vi "MergeFilesManual.vi"(4 "Error In":errorcluster, 7 "MergeFileConfINPUT":T1) -> (0 "sortie d'erreur":errorcluster)   [LabVIEW 2017]
uses:
  DefDeType/MergeFileConfig.ctl
  DefDeType/WhichPath.ctl
panel:
  out "MergeFileConfig":T1
  in  "Cancel":bool
  in  "OK Merge":bool
  out "AllWaveForms":waveform(dbl)[](graph)
  out "QUALISYSWaveForms":waveform(dbl)[](graph)
  out "HBMWaveform":waveform(dbl)[](graph)
  out "PCIWaveforms":waveform(dbl)[](graph)
  out "Etat":string
  # "Merging files"
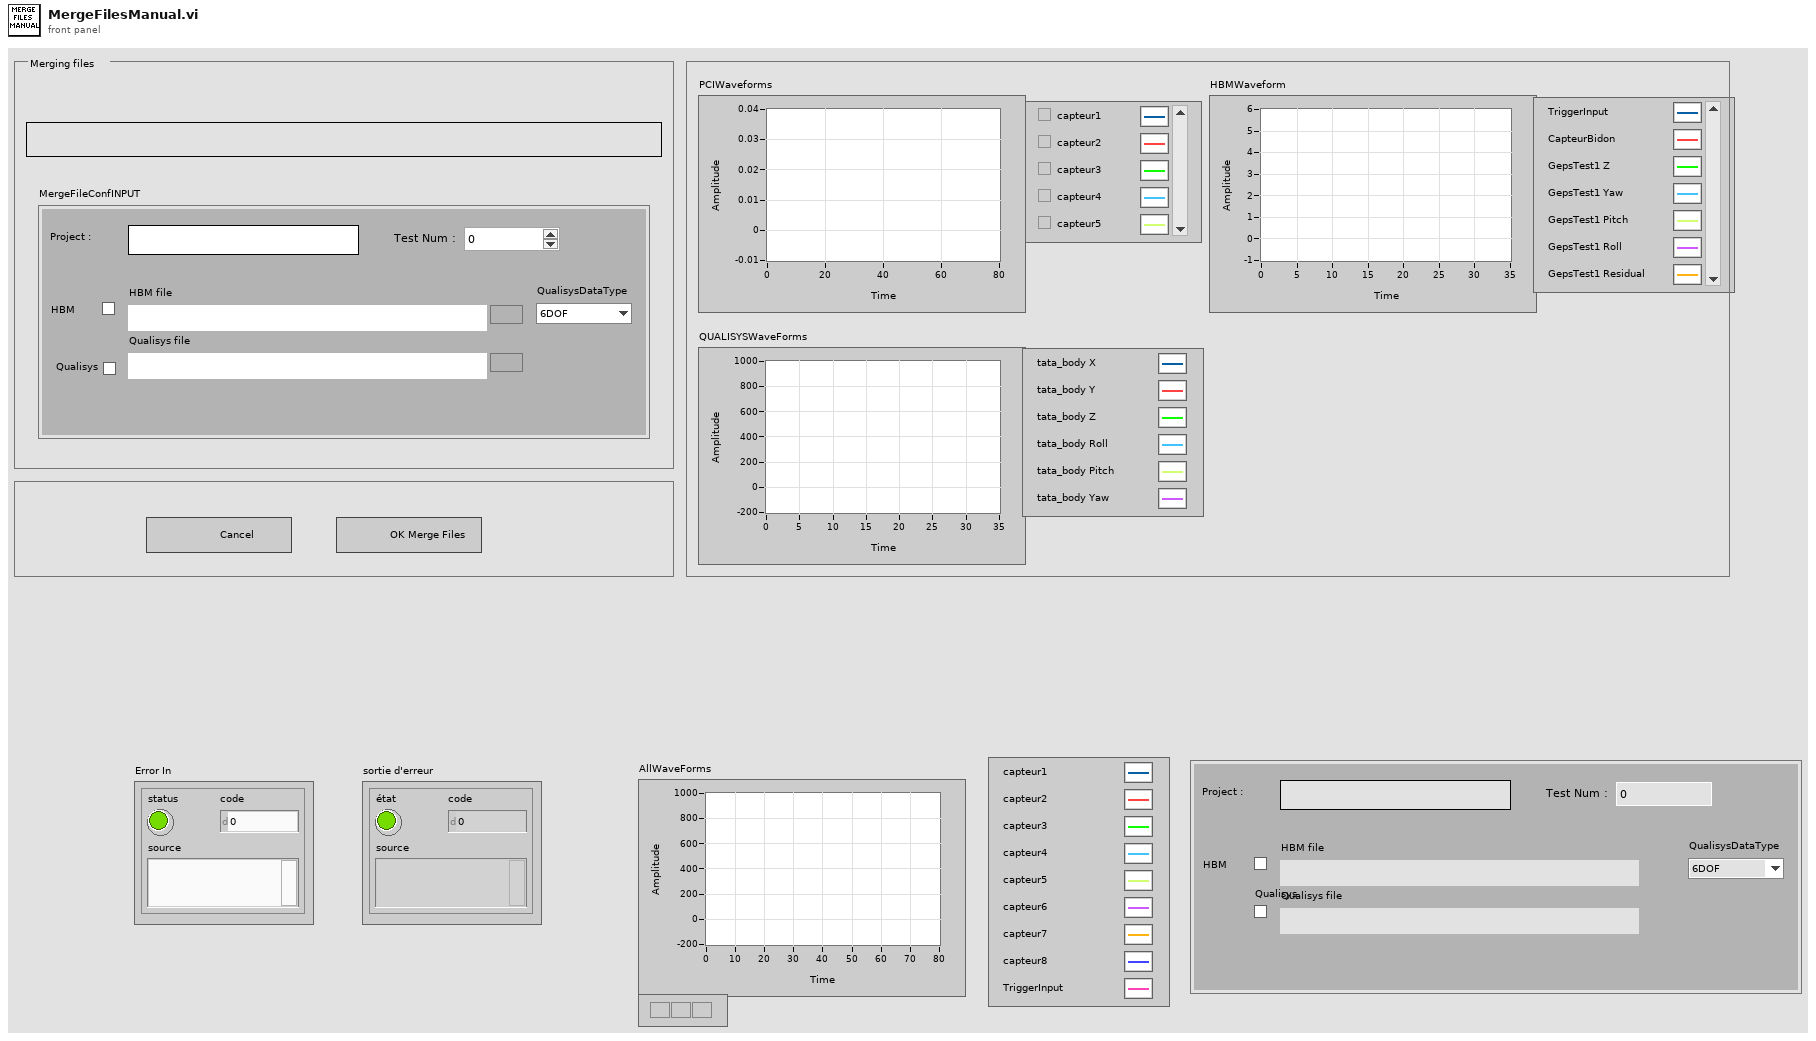
[diagram p1: front panel]
types:
  T1 = typedef "MergeFileConfig.ctl" = cluster{"Test Num : ":u32, "Project :":string, "Qualisys file":path, "HBM file":path, "QualisysDataType":enum16{"6DOF", "3DTracking", "6DOF + 3D"}, "Qualisys":bool, "HBM":bool}
  T2 = enum16{"open", "open or create", "create or replace", "create", "open (read-only)"}
  T3 = typedef "WhichPath.ctl" = enum16{"DossierProjet", "Config", "Meas", "MeasPCI", "MeasCRIO1", "MeasCRIO2", "MeasQualisys", "MeasHBM", "MeasTDMS", "Fig", "Res"}
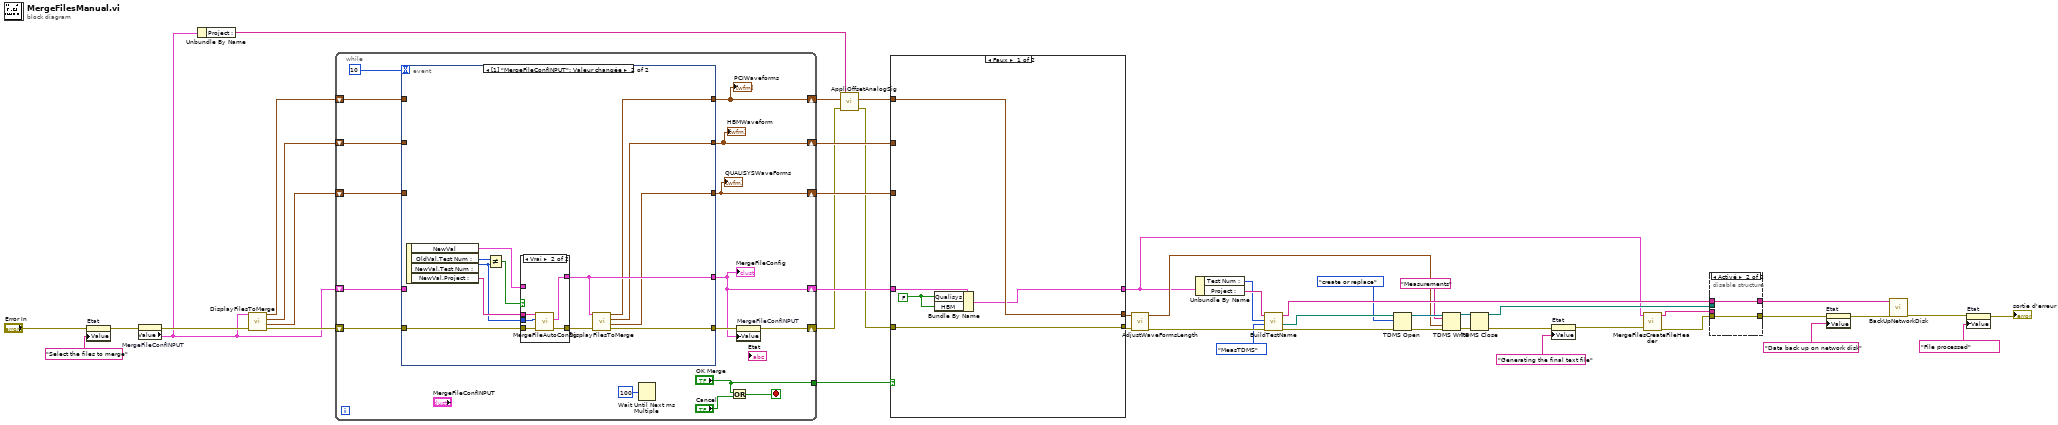
[diagram p0: block diagram]
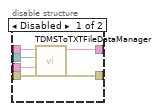
[diagram p2: hidden frame]
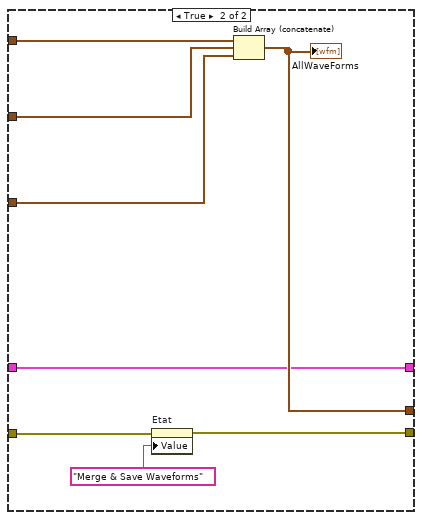
[diagram p3: hidden frame]
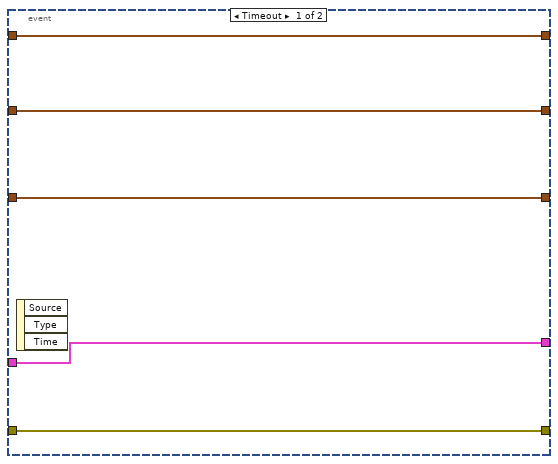
[diagram p4: hidden frame]
diagram:
  n1 = property on="Etat" class="Ch"(error in="Error In", "Value"="Select the files to merge" ("Etat")) -> (error out=w10:errorcluster)  [unwired: 1 in, 1 out]
  n2 = property on="MergeFileConfINPUT" class="Clust (strict)"(error in=w10) -> (error out=w9:errorcluster, "Value"=w4:T1)  [unwired: 1 in, 1 out]
  n3 = Unbundle By Name(w4) -> ("Project :"=w3:string)
  n4 = call "DisplayFilesToMerge.vi"("Error In"=w9, "MergeFileConfigIN"=w4) -> ("Error Out"=w45:errorcluster, "QualisysWaveform"=w1:waveform(dbl)[], "HBMWaveForms"=w2:waveform(dbl)[], "PCIWaveform"=w44:waveform(dbl)[])  [unwired: 2 in]
  n5 = while {
    shift-right: [w57] -> w8
    shift-left: w44 -> [w60]
    shift-right: [w56] -> w46
    shift-left: w2 -> [w59]
    shift-right: [w55] -> w47
    shift-left: w1 -> [w58]
    shift-right: [w51] -> w6
    shift-left: w45 -> [w54]
    tunnel: ["OK Merge"] -> w14
    shift-right: [w49] -> w13
    shift-left: w4 -> [w52]
    stop <- w63 stop-if-true
    n6 = event shown="[1] \"MergeFileConfINPUT\": Valeur changée" {
      selector: _ -> [_ _]
      dyn-events: _ -> [_ _]
      timeout: 10 -> [_ _]
      tunnel: w60 -> [w69 _]
      tunnel: w59 -> [w68 _]
      tunnel: w58 -> [w67 _]
      tunnel: [w69 w72] -> w57
      tunnel: [w68 w71] -> w56
      tunnel: [w67 w70] -> w55
      tunnel: w54 -> [w66 w78]
      tunnel: [w66 w81] -> w50
      tunnel: w52 -> [w65 _]
      tunnel: [w65 w73] -> w49
      event Timeout {
        n7 = event-data() -> ()  [unwired: 1 in, 3 out]
      }
      event Value Change {
        n8 = event-data() -> ("NewVal"=w74:T1, "OldVal.Test Num :"=w80:u32, "NewVal.Test Num :"=w75:u32, "NewVal.Project :"=w77:string)  [unwired: 1 in]
        n9 = Not Equal?(x=w80, y=w75) -> (x != y?=w76:bool)
        n10 = case shown="Vrai" w76 {
          tunnel: [w83 w87] -> w79
          tunnel: w78 -> [w83 w88]
          tunnel: w77 -> [_ w86]
          tunnel: w75 -> [_ w85]
          tunnel: w74 -> [w82 _]
          tunnel: [w82 w84] -> w73
          frame False {
          }
          frame True {
            n11 = call "MergeFileAutoConfig.vi"("error in (no error)"=w88, "test num"=w85, "ProjetIN"=w86) -> ("error out"=w87:errorcluster, "MergeFileConfigOUT"=w84:T1)  [unwired: 2 in, 1 out]
          }
        }
        n12 = call "DisplayFilesToMerge.vi"("Error In"=w79, "MergeFileConfigIN"=w73) -> ("Error Out"=w81:errorcluster, "QualisysWaveform"=w70:waveform(dbl)[], "HBMWaveForms"=w71:waveform(dbl)[], "PCIWaveform"=w72:waveform(dbl)[])  [unwired: 2 in]
      }
    }
    "PCIWaveforms" <- w57
    "HBMWaveform" <- w56
    "QUALISYSWaveForms" <- w55
    "MergeFileConfig" <- w49
    n13 = Wait Until Next ms Multiple(millisecond multiple=u32 100) -> ()  [unwired: 1 out]
    n14 = Or(x="OK Merge", y="Cancel") -> (x .or. y?=w63:bool)
    n15 = property on="MergeFileConfINPUT" class="Clust (strict)"(error in=w50, "Value"=w49) -> (error out=w51:errorcluster)  [unwired: 1 in, 1 out]
  }
  n16 = call "AppliOffsetAnalogSig.vi"("error in (no error)"=w6, "WaveFormIN"=w8, "NomProjet"=w3) -> ("error out"=w5:errorcluster, "WaveFormOUT"=w7:waveform(dbl)[])  [unwired: 3 in]
  n17 = case shown="Faux" w14 {
    tunnel: w47 -> [_ w101]
    tunnel: w46 -> [_ w100]
    tunnel: w7 -> [w92 w99]
    tunnel: w5 -> [w93 w98]
    tunnel: [w92 w97] -> w24
    tunnel: [w93 w95] -> w22
    tunnel: w13 -> [w91 w94]
    tunnel: [w90 w94] -> w12
    frame False {
      w89 = FALSE ("Qualisys")
      n18 = Bundle By Name(cluster=w91, "Qualisys"=w89, "HBM"=w89) -> (w90:T1)
    }
    frame True {
      n19 = property on="Etat" class="Ch"(error in=w98, "Value"="Merge & Save Waveforms" ("Etat")) -> (error out=w95:errorcluster)  [unwired: 1 in, 1 out]
      n20 = Build Array (concatenate)(w99, w100, w101) -> (w97:waveform(dbl)[])
      "AllWaveForms" <- w97
    }
  }
  n21 = call "AdjustWaveFormsLength.vi"("error in (no error)"=w22, "AllWaveFormsIN"=w24) -> ("error out"=w34:errorcluster, "AllWaveFormsOUT"=w20:waveform(dbl)[])  [unwired: 4 in]
  n22 = Unbundle By Name(w12) -> ("Test Num :"=w18:u32, "Project :"=w19:string)
  n23 = call "BuildTestName.vi"("entrée d'erreur"=w34, "WhichPath?"=WhichPath."MeasTDMS", "NextTestNum"=w18, "NomProjet"=w19) -> ("sortie d'erreur"=w31:errorcluster, "cheminProchainFichier"=w28:path, "NomProjetOut"=w33:string)  [unwired: 1 in, 1 out]
  n24 = TDMS Open(8:w31, 10:T2."create or replace" ("operation (0:open)"), 11:w28) -> (0:w30:errorcluster, 3:w26:refnum<k34>)  [unwired: 4 in]
  n25 = TDMS Write(0:w26, 5:"Measurements" ("group name in (Untitled)"), 9:w20, 11:w30) -> (4:w25:refnum<k34>, 15:w29:errorcluster)  [unwired: 2 in, 2 out]
  n26 = TDMS Close(8:w29, 11:w25) -> (0:w23:errorcluster, 3:w21:path)
  n27 = property on="Etat" class="Ch"(error in=w23, "Value"="Generating the final text file" ("Etat")) -> (error out=w17:errorcluster)  [unwired: 1 in, 1 out]
  n28 = call "MergeFilesCreateFileHeader.vi"("Error In"=w17, "MergeFileConfig"=w12) -> ("Error Out"=w16:errorcluster, "TextFileHeader"=w15:string)  [unwired: 4 in]
  n29 = disable-structure shown="Activé" {
    disable-tunnel: [w107 w108] -> w38
    disable-tunnel: [w106 w109] -> w37
    disable-tunnel: w33 -> [w105 w109]
    disable-tunnel: w21 -> [w104 _]
    disable-tunnel: w16 -> [w103 w108]
    disable-tunnel: w15 -> [w102 _]
    frame Disabled {
      n30 = call "TDMSToTXTFileDataManager.vi"("entrée d'erreur"=w103, "Info(analog acq,wave,Quali,hexap...)"=w102, "FichierTDMSOrigine"=w104, "NomProj"=w105) -> ("sortie d'erreur"=w107:errorcluster, "NomProjOUT"=w106:string)  [unwired: 1 in, 1 out]
    }
    frame Enabled {
    }
  }
  n31 = property on="Etat" class="Ch"(error in=w38, "Value"="Data back up on network disk" ("Etat")) -> (error out=w39:errorcluster)  [unwired: 1 in, 1 out]
  n32 = call "BackUpNetworkDisk.vi"("Entrée d'erreur"=w39, "NomProjet"=w37) -> ("error out"=w36:errorcluster)  [unwired: 2 in, 1 out]
  n33 = property on="Etat" class="Ch"(error in=w36, "Value"="File processed" ("Etat")) -> (error out=→"sortie d'erreur":errorcluster)  [unwired: 1 in, 1 out]
